vi "Actor Core.vi"(8 "error in":errorcluster, 11 "Panel Form Controller in":refnum<class "Panel Form Controller.lvclass">) -> (0 "error out":errorcluster, 3 "Actor out":refnum<class "Actor.lvclass">)   [LabVIEW 2020, in "Panel Form Controller.lvlib" / "Panel Form Controller.lvclass"]
doc: "The user interface for this panel.\n\n----\nPlease see the following web address for additional documentation and tutorial information:\nhttp://www.mooregoodideas.com/mgi-panel-manager/\n\nAuthor: Derek Trepanier\n\nCopyright (c) 2018, Moore Good Ideas, Inc.\n\nAll rights reserved.\n\nRedistribution and use in source and binary forms, with or without modification, are permitted provided that the following conditions are met:\n\n * Redistributions of source code must retain the above copyright notice, this list of conditions and the following disclaimer.\n * Redistributions in binary form must reproduce the above copyright notice, this list of conditions and the following disclaimer in the documentation and/or other materials provided with the distribution.\n * Neither the name of Moore Good Ideas, Inc. nor the names of its contributors may be used to endorse or promote products derived from this software without specific prior written permission.\n\nTHIS SOFTWARE IS PROVIDED BY THE COPYRIGHT HOLDERS AND CONTRIBUTORS \"AS IS\" AND ANY EXPRESS OR IMPLIED WARRANTIES, INCLUDING, BUT NOT LIMITED TO, THE IMPLIED WARRANTIES OF MERCHANTABILITY AND FITNESS FOR A PARTICULAR PURPOSE ARE DISCLAIMED. IN NO EVENT SHALL THE COPYRIGHT OWNER OR CONTRIBUTORS BE LIABLE FOR ANY DIRECT, INDIRECT, INCIDENTAL, SPECIAL, EXEMPLARY, OR CONSEQUENTIAL DAMAGES (INCLUDING, BUT NOT LIMITED TO, PROCUREMENT OF SUBSTITUTE GOODS OR SERVICES; LOSS OF USE, DATA, OR PROFITS; OR BUSINESS INTERRUPTION) HOWEVER CAUSED AND ON ANY THEORY OF LIABILITY, WHETHER IN CONTRACT, STRICT LIABILITY, OR TORT (INCLUDING NEGLIGENCE OR OTHERWISE) ARISING IN ANY WAY OUT OF THE USE OF THIS SOFTWARE, EVEN IF ADVISED OF THE POSSIBILITY OF SUCH DAMAGE."
uses:
  Panel Form Controller.lvclass
  C:/Program Files (x86)/National Instruments/LabVIEW 2020/vi.lib/MGI/Panel Manager/Panel Actor/Panel Actor/Panel Actor.lvclass
  <vilib>/ActorFramework/Actor/Actor.lvclass
  <vilib>/MGI/Panel Manager/Panel/Panel Helper/Panel Events.ctl
  <vilib>/MGI/Panel Manager/Panel/Panel Helper/Events.ctl
  <vilib>/ActorFramework/Message Enqueuer/Message Enqueuer.lvclass/Message Enqueuer.ctl
  <vilib>/ActorFramework/Message Enqueuer/Enqueue.vi
  <vilib>/ActorFramework/Stop Msg/Stop Msg.lvclass
  C:/Program Files (x86)/National Instruments/LabVIEW 2020/vi.lib/ActorFramework/Message/Message.lvclass
  <vilib>/ActorFramework/Message Priority Queue/Priority Enqueue.vi
  <vilib>/MGI/Panel Manager/Panel Actor/Panel Actor/Panel Actor.lvclass
  <vilib>/MGI/Panel Manager/Panel/Panel Helper/Panel Helper.lvclass
types:
  T1 = cluster{"Pnl Actor":refnum<event-registration>, "Child Pnl":refnum<event-registration>, "Child Fields":refnum<event-registration>, "Child Buttons":refnum<event-registration>}
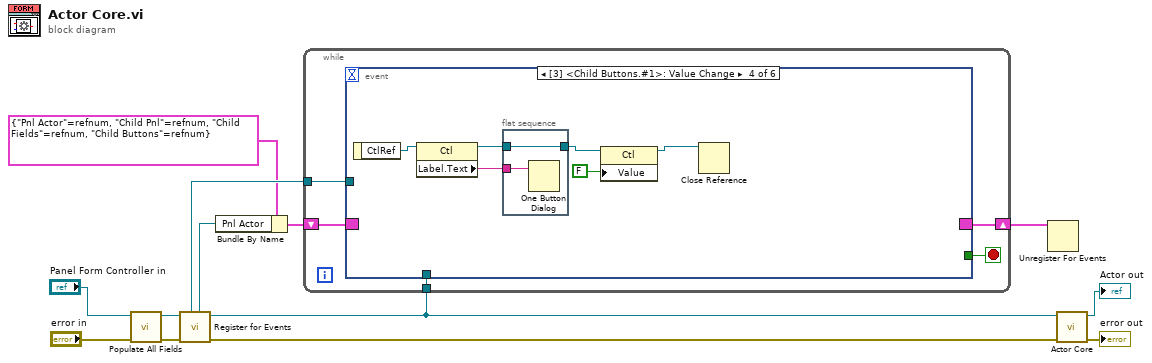
[diagram p0: block diagram]
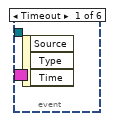
[diagram p2: hidden frame]
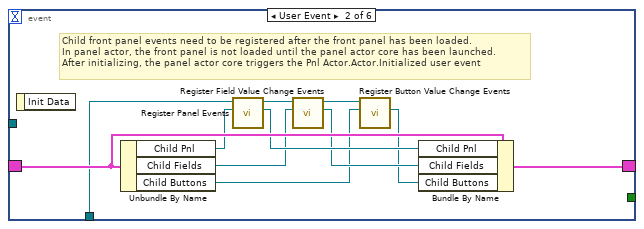
[diagram p3: hidden frame]
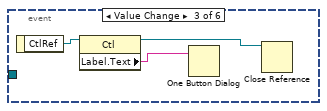
[diagram p4: hidden frame]
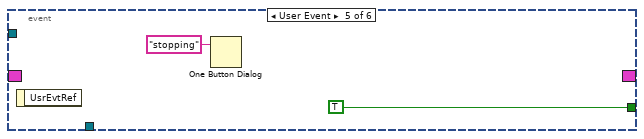
[diagram p5: hidden frame]
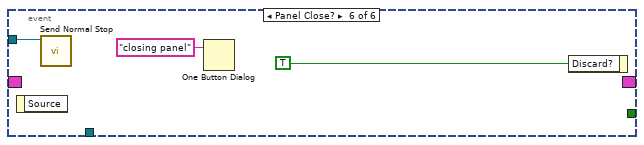
[diagram p6: hidden frame]
diagram:
  n1 = call "Populate All Fields.vi"("error in (no error)"="error in", "Panel Form Controller in"="Panel Form Controller in") -> ("error out"=w1:errorcluster, "Panel Form Controller out"=w3:refnum<class "Panel Form Controller.lvclass">)  [unwired: 8 in]
  n2 = call <vilib>:"Register for Events.vi"("Error In"=w1, "Panel Actor in"=w3) -> ("Error Out"=w6:errorcluster, "Panel Actor out"=w5:refnum<class "Panel Form Controller.lvclass">, "Pnl Actor"=w7:refnum<event-registration>, "Self Enqueuer"=w10:refnum<class "Message Enqueuer.lvclass">)  [unwired: 6 in]
  n3 = Bundle By Name(cluster=T1 {"Pnl Actor"=refnum, "Child Pnl"=refnum, "Child Fields"=refnum, "Child Buttons"=refnum}, "Pnl Actor"=w7) -> (w8:T1)
  n4 = while {
    tunnel: w10 -> [w18]
    tunnel: w5 -> [w14]
    shift-right: [w16] -> w11
    shift-left: w8 -> [w15]
    stop <- w17 stop-if-true
    n5 = event shown="[3] <Child Buttons.#1>: Value Change" {
      selector: w15 -> [_ w29 _ _ _ _]
      dyn-events: [_ w28 _ _ _ _] -> w16
      timeout: _ -> [_ _ _ _ _ _]
      tunnel: w18 -> [_ _ _ _ _ w45]
      tunnel: [_ _ _ _ TRUE _] -> w17
      tunnel: w14 -> [_ w22 _ _ _ _]
      event Timeout {
        n6 = event-data() -> ()  [unwired: 1 in, 3 out]
      }
      event User Event {
        # "Child front panel events need to be registered after the front panel has been loaded.\nIn panel actor, the front panel is not loaded until the panel actor core has been launched.\nAfter initializing, the panel actor core triggers the Pnl Actor.Actor.Initialized user event"
        n7 = event-data() -> ()  [unwired: 1 in, 1 out]
        n8 = Unbundle By Name(w29) -> ("Child Pnl"=w27:refnum<event-registration>, "Child Fields"=w25:refnum<event-registration>, "Child Buttons"=w20:refnum<event-registration>)
        n9 = call "Register Panel Events.vi"("Event Refnum In"=w27, "Panel Form Controller in"=w22) -> ("Event Refnum Out"=w26:refnum<event-registration>, "Panel Form Controller out"=w23:refnum<class "Panel Form Controller.lvclass">)  [unwired: 7 in, 1 out]
        n10 = call "Register Field Value Change Events.vi"("Field Event Refnum In"=w25, "Panel Form Controller in"=w23) -> ("Field Event Refnum Out"=w24:refnum<event-registration>, "Panel Form Controller out"=w21:refnum<class "Panel Form Controller.lvclass">)  [unwired: 7 in, 1 out]
        n11 = call "Register Button Value Change Events.vi"("Button Event Refnum In"=w20, "Panel Form Controller in"=w21) -> ("Button Event Refnum Out"=w19:refnum<event-registration>)  [unwired: 7 in, 2 out]
        n12 = Bundle By Name(cluster=w29, "Child Pnl"=w26, "Child Fields"=w24, "Child Buttons"=w19) -> (w28:T1)
      }
      event Value Change {
        n13 = event-data() -> ("CtlRef"=w32:refnum<vi>)  [unwired: 1 in]
        n14 = property class="Ctl"(reference=w32) -> (reference out=w30:refnum<vi>, "Label.Text"=w31:string)  [unwired: 1 in, 1 out]
        n15 = One Button Dialog(message=w31) -> ()  [unwired: 1 in, 1 out]
        n16 = Close Reference(reference=w30) -> ()  [unwired: 1 in, 1 out]
      }
      event Value Change {
        n17 = event-data() -> ("CtlRef"=w38:refnum<vi>)  [unwired: 1 in]
        n18 = property class="Ctl"(reference=w38) -> (reference out=w34:refnum<vi>, "Label.Text"=w37:string)  [unwired: 1 in, 1 out]
        n19 = flat-sequence {
          tunnel: w37 -> [w40]
          tunnel: w34 -> [w39]
          tunnel: [w39] -> w33
          frame #0 {
            n20 = One Button Dialog(message=w40) -> ()  [unwired: 1 in, 1 out]
          }
        }
        n21 = property class="Ctl"(reference=w33, "Value"=FALSE) -> (reference out=w36:refnum<vi>)  [unwired: 1 in, 1 out]
        n22 = Close Reference(reference=w36) -> ()  [unwired: 1 in, 1 out]
      }
      event User Event {
        n23 = event-data() -> ()  [unwired: 1 in, 1 out]
        n24 = One Button Dialog(message="stopping") -> ()  [unwired: 1 in, 1 out]
      }
      event Panel Close? {
        n25 = event-data() -> ()  [unwired: 1 in, 1 out]
        n26 = call <vilib>:"Send Normal Stop.vi"("Message Enqueuer"=w45) -> ()  [unwired: 10 in, 1 out]
        n27 = One Button Dialog(message="closing panel") -> ()  [unwired: 1 in, 1 out]
        n28 = event-data("Discard?"=TRUE) -> ()  [unwired: 1 in, 1 out]
      }
    }
  }
  n29 = Unregister For Events(event registration refnum=w11) -> ()  [unwired: 1 in, 1 out]
  n30 = call-parent "Actor Core.vi"("error in"=w6, "Panel Actor in"=w5) -> ("error out"=→"error out":errorcluster, "Actor out"=→"Actor out":refnum<class "Actor.lvclass">)  [unwired: 8 in]
